vi "InitFromXML.vi"(8 "error in (no error)":errorcluster, 10 "XML":string, 11 "RingItemVINoParams in":refnum<class "RingItemVINoParams.lvclass">) -> (0 "error out":errorcluster, 3 "RingItemVINoParams out":refnum<class "RingItemVINoParams.lvclass">)   [LabVIEW 2009, in "NavScreen.lvlib" / "RingItemVINoParams.lvclass"]
uses:
  RingItemVINoParams.lvclass
  RingItem/RingItem.lvclass
  RingItemVINoParams.lvclass/RingItemVINoParams.ctl
  NavScreen.lvlib
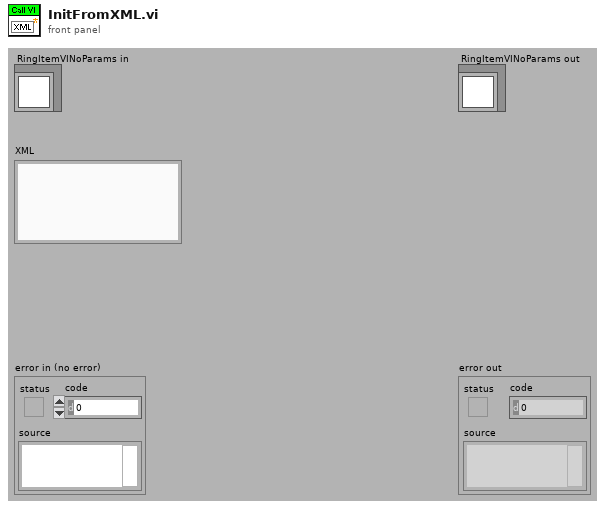
[diagram p1: front panel]
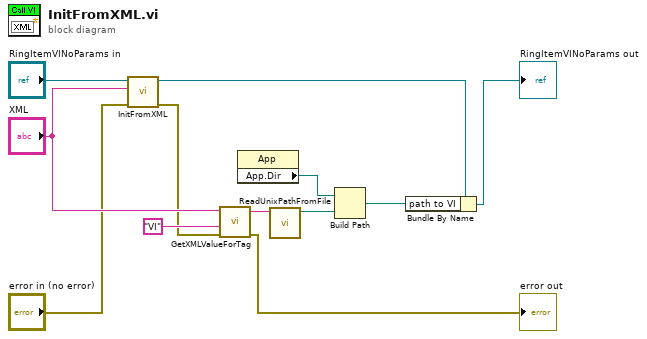
[diagram p0: block diagram]
diagram:
  n1 = call-parent "InitFromXML.vi"("error in (no error)"="error in (no error)", "XML"="XML", "RingItem in"="RingItemVINoParams in") -> ("error out"=w8:errorcluster, "RingItem out"=w4:refnum<class "RingItemVINoParams.lvclass">)  [unwired: 7 in]
  n2 = call "GetXMLValueForTag.vi"("error in (no error)"=w8, "tag"="VI", "XML"="XML") -> ("error out"=→"error out":errorcluster, "value"=w7:string)  [unwired: 7 in]
  n3 = property class="App"() -> ("App.Dir"=w6:path)  [unwired: 2 in, 2 out]
  n4 = call "ReadUnixPathFromFile.vi"("path"=w7) -> ("path"=w5:path)  [unwired: 10 in]
  n5 = Build Path(base path=w6, name or relative path=w5) -> (appended path=w3:path)
  n6 = Bundle By Name(cluster=w4, "path to VI"=w3) -> (→"RingItemVINoParams out":refnum<class "RingItemVINoParams.lvclass">)
